vi "Dequeue Message.vi"(8 "error in (no error)":errorcluster) -> (0 "error out":errorcluster, 2 "Element":T1)   [LabVIEW 2020, in "Display Console.lvlib"]
doc: "This VI pulls messages off the Message Queue."
uses:
  Display Console.lvlib
  Private Controls/Message Cluster.ctl
  Private Controls/Message enum.ctl
  Private Controls/FG Actions.ctl
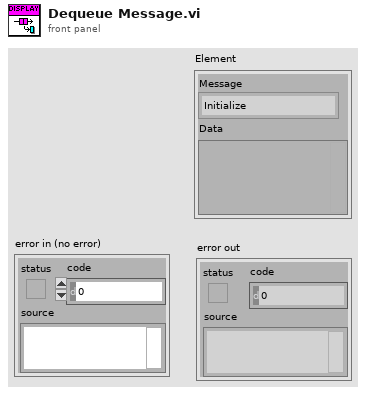
[diagram p1: front panel]
types:
  T1 = typedef "Display Console.lvlib/Message Cluster.ctl" = cluster{"Message":T2, "Data":variant}
  T2 = typedef "Display Console.lvlib/Message enum.ctl" = enum16{"Initialize", "Update Message", "Terminate State", "Error", "Exit"}
  T3 = typedef "Display Console.lvlib/FG Actions.ctl" = enum16{"Get", "Set", "Clear"}
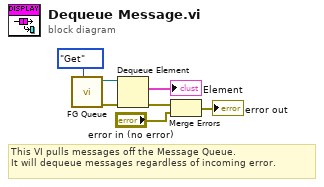
[diagram p0: block diagram]
diagram:
  # "This VI pulls messages off the Message Queue.\nIt will dequeue messages regardless of incoming error."
  n1 = call "FG Queue.vi"("FG Actions"=FG_Actions."Get") -> ("error out"=w3:errorcluster, "Message Queue Out"=w4:refnum<queue>)  [unwired: 9 in]
  n2 = Dequeue Element(queue=w4, error in (no error)=w3) -> (element=→"Element":T1, error out=w6:errorcluster)  [unwired: 1 in, 2 out]
  n3 = Merge Errors(w6, "error in (no error)") -> (→"error out":errorcluster)
